vi "Check.vi"(8 "Error In":errorcluster, 10 "Result":refnum<class "IResult.lvclass">, 11 "AlarmIn":refnum<class "IAlarm.lvclass">) -> (0 "Error Out":errorcluster, 2 "Raised?":bool, 3 "AlarmOut":refnum<class "IAlarm.lvclass">)   [LabVIEW 2019, in "IAlarm.lvclass"]
uses:
  IAlarm.lvclass
  IResult/IResult.lvclass
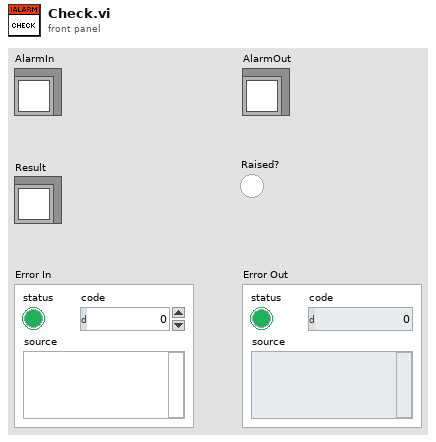
[diagram p1: front panel]
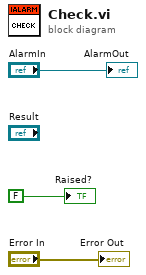
[diagram p0: block diagram]
diagram:
  "AlarmOut" <- "AlarmIn"
  "Error Out" <- "Error In"
  "Raised?" <- FALSE ("Raised?")
